vi "EX2.vi"() -> ()   [LabVIEW 2024]
panel:
  out "String":string
  out "Boolean":bool
  out "Boolean 4":bool
  out "Boolean 3":bool
  out "carreau gris":dbl(slide) scale=0.0..10.0
  out "Slide 5":dbl(slide) scale=0.0..10.0
  out "carreau bleu":dbl(slide) scale=0.0..10.0
  out "Slide 4":dbl(slide) scale=0.0..10.0
  out "meche drill":dbl(slide) scale=0.0..10.0
  out "time string":string
  out "date string":string
  out "COMPTAGE PIECES":dbl
  in  "Boolean 2":bool
  # "TP N°1"
  # "Mekni Marwen 2ème Année Génie Electrique"
  # "Exercice 2 : Perceuse"
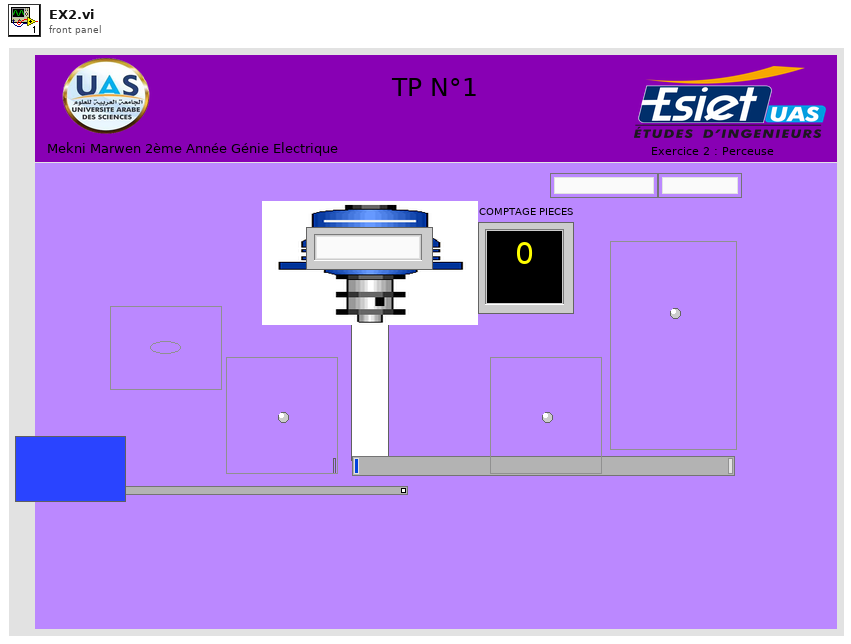
[diagram p1: front panel]
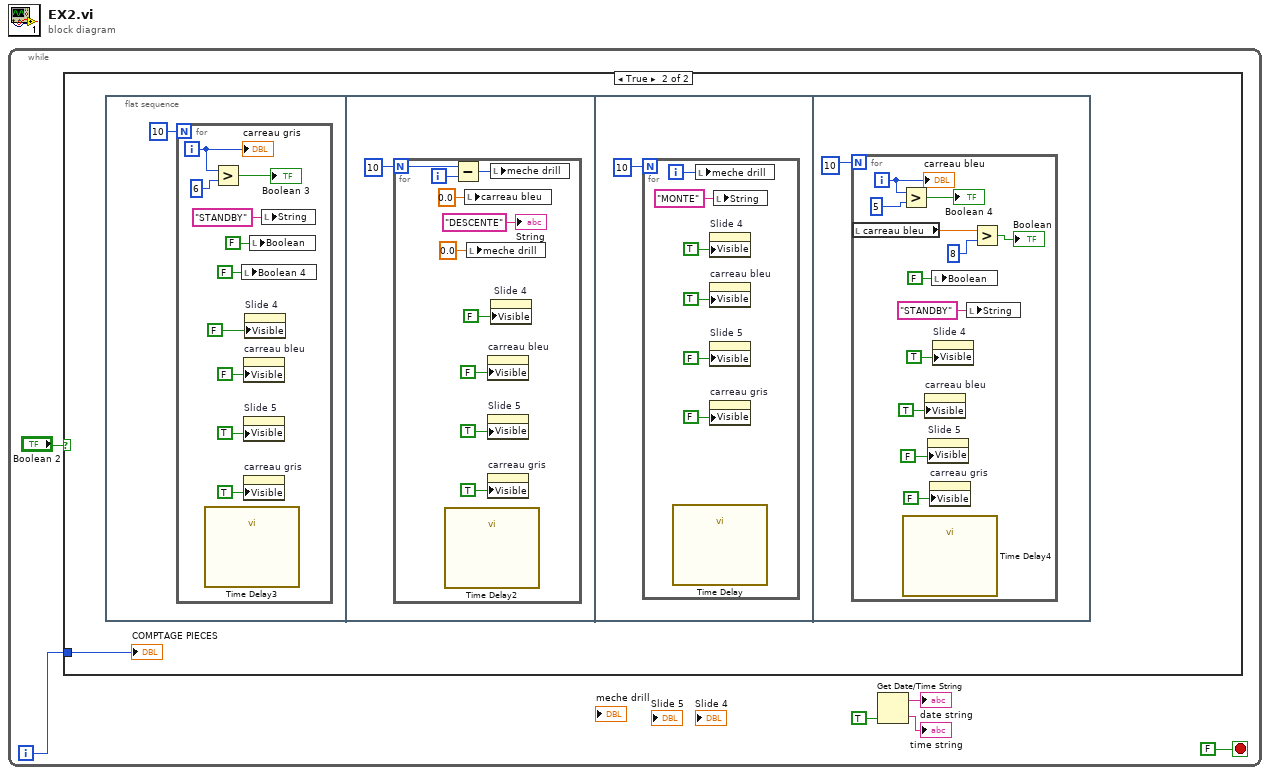
[diagram p0: block diagram]
diagram:
  n1 = while {
    i -> [w1]
    stop <- FALSE stop-if-true
    n2 = case shown="True" "Boolean 2" {
      tunnel: w1 -> [_ w7]
      frame False {
      }
      frame True {
        n3 = flat-sequence {
          frame #0 {
            n4 = for {
              N: 10 -> [_]
              i -> [w14]
              n5 = call "Time Delay3"() -> ()  [unwired: 11 in, 1 out]
              n6 = Greater?(x=w14, y=6) -> (0:→"Boolean 3":bool)
              n7 = local write "Boolean 4"(FALSE ("Boolean 4")) -> ()
              n8 = property on="carreau bleu" class="Slide (strict)"("Visible"=FALSE) -> ()  [unwired: 2 in, 2 out]
              n9 = property on="Slide 5" class="Slide (strict)"("Visible"=TRUE) -> ()  [unwired: 2 in, 2 out]
              n10 = property on="carreau gris" class="Slide (strict)"("Visible"=TRUE) -> ()  [unwired: 2 in, 2 out]
              n11 = property on="Slide 4" class="Slide (strict)"("Visible"=FALSE) -> ()  [unwired: 2 in, 2 out]
              n12 = local write "Boolean"(FALSE ("Boolean")) -> ()
              n13 = local write "String"("STANDBY" ("String")) -> ()
              "carreau gris" <- w14
            }
          }
          frame #1 {
            n14 = for {
              N: 10 -> [w29]
              i -> [w28]
              n15 = call "Time Delay2"() -> ()  [unwired: 11 in, 1 out]
              n16 = Subtract(x=w29, y=w28) -> (x-y=w27:i32)
              n17 = local write "carreau bleu"(0.0 ("carreau bleu")) -> ()
              n18 = local write "meche drill"(0.0 ("meche drill")) -> ()
              n19 = property on="carreau bleu" class="Slide (strict)"("Visible"=FALSE) -> ()  [unwired: 2 in, 2 out]
              n20 = property on="Slide 5" class="Slide (strict)"("Visible"=TRUE) -> ()  [unwired: 2 in, 2 out]
              n21 = property on="carreau gris" class="Slide (strict)"("Visible"=TRUE) -> ()  [unwired: 2 in, 2 out]
              n22 = local write "meche drill"(w27) -> ()
              n23 = property on="Slide 4" class="Slide (strict)"("Visible"=FALSE) -> ()  [unwired: 2 in, 2 out]
              "String" <- "DESCENTE" ("String")
            }
          }
          frame #2 {
            n24 = for {
              N: 10 -> [_]
              i -> [w36]
              n25 = call "Time Delay"() -> ()  [unwired: 11 in, 1 out]
              n26 = local write "meche drill"(w36) -> ()
              n27 = property on="Slide 4" class="Slide (strict)"("Visible"=TRUE) -> ()  [unwired: 2 in, 2 out]
              n28 = property on="carreau bleu" class="Slide (strict)"("Visible"=TRUE) -> ()  [unwired: 2 in, 2 out]
              n29 = property on="Slide 5" class="Slide (strict)"("Visible"=FALSE) -> ()  [unwired: 2 in, 2 out]
              n30 = property on="carreau gris" class="Slide (strict)"("Visible"=FALSE) -> ()  [unwired: 2 in, 2 out]
              n31 = local write "String"("MONTE" ("String")) -> ()
            }
          }
          frame #3 {
            n32 = for {
              N: 10 -> [_]
              i -> [w43]
              n33 = local read "carreau bleu"() -> (w40:dbl)
              n34 = Greater?(x=w43, y=5) -> (0:→"Boolean 4":bool)
              n35 = call "Time Delay4"() -> ()  [unwired: 11 in, 1 out]
              n36 = property on="carreau bleu" class="Slide (strict)"("Visible"=TRUE) -> ()  [unwired: 2 in, 2 out]
              n37 = property on="Slide 5" class="Slide (strict)"("Visible"=FALSE) -> ()  [unwired: 2 in, 2 out]
              n38 = property on="carreau gris" class="Slide (strict)"("Visible"=FALSE) -> ()  [unwired: 2 in, 2 out]
              n39 = local write "Boolean"(FALSE ("Boolean")) -> ()
              n40 = property on="Slide 4" class="Slide (strict)"("Visible"=TRUE) -> ()  [unwired: 2 in, 2 out]
              n41 = local write "String"("STANDBY" ("String")) -> ()
              n42 = Greater?(x=w40, y=8) -> (0:→"Boolean":bool)
              "carreau bleu" <- w43
            }
          }
        }
        "COMPTAGE PIECES" <- w7
      }
    }
    n43 = Get Date/Time String(want seconds? (F)=TRUE) -> (date string=→"date string":string, time string=→"time string":string)  [unwired: 2 in]
  }
